vi "Write Skills.vi"(8 "error in (no error)":errorcluster, 10 "Skills":refnum<class "Skill_v2.lvclass">[](array[class]), 11 "Tactic_v2 in":refnum<class "Tactic_v2.lvclass">) -> (0 "error out":errorcluster, 3 "Tactic_v2 out":refnum<class "Tactic_v2.lvclass">)   [LabVIEW 2023, in "Tactic_v2.lvclass"]
uses:
  Tactic_v2.lvclass
  NewSkills/Skill_v2_class/Skill_v2.lvclass
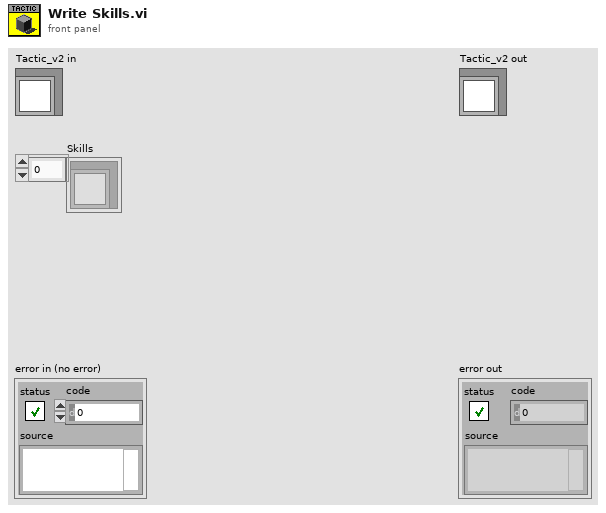
[diagram p1: front panel]
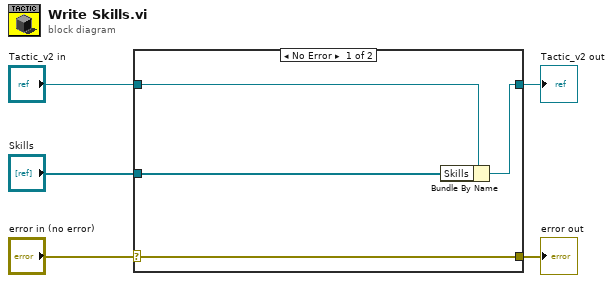
[diagram p0: block diagram]
diagram:
  n1 = case shown="No Error" "error in (no error)" {
    selector: "error in (no error)" -> [w9 w10]
    tunnel: [w9 w10] -> w4
    tunnel: [w7 w11] -> w2
    tunnel: "Tactic_v2 in" -> [w8 w11]
    tunnel: "Skills" -> [w6 _]
    frame No Error {
      n2 = Bundle By Name(cluster=w8, "Skills"=w6) -> (w7:refnum<class "Tactic_v2.lvclass">)
    }
    frame Error {
    }
  }
  "error out" <- w4
  "Tactic_v2 out" <- w2
